vi "Main_Timing.vi"() -> ()   [LabVIEW 2012]
panel:
  in  "Wait between operations (ms)":dbl
  in  "Input Expression":string
  out "While Iterations":i32
  out "Elapsed Time (ms)":dbl caption="Elapsed Time (s)"
  in  "Time Target (ms)":dbl=5.0 caption="Time Target (s)"
  # "(5 operations)"
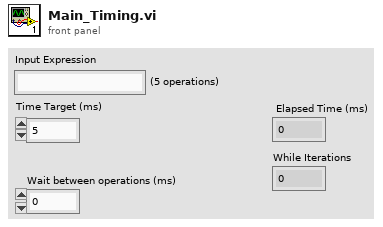
[diagram p1: front panel]
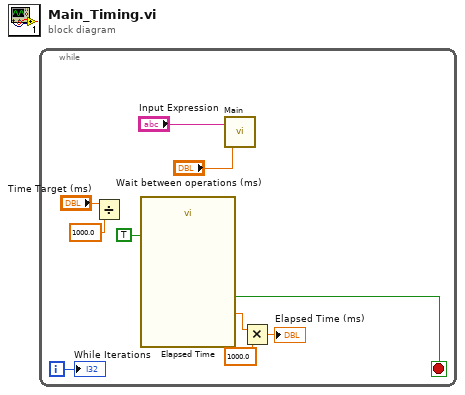
[diagram p0: block diagram]
diagram:
  n1 = while {
    i -> [w8]
    stop <- w9 stop-if-true
    n2 = Divide(x="Time Target (ms)", y=1000.0) -> ()  [unwired: 1 out]
    n3 = call "Elapsed Time"("Auto Reset"=TRUE) -> ("Elapsed Time (s)"=w3:dbl, "Time has Elapsed"=w9:bool)  [unwired: 11 in, 6 out]
    n4 = call "Main.vi"("Wait (ms)"="Wait between operations (ms)", "Input Expression"="Input Expression") -> ()  [unwired: 1 out]
    n5 = Multiply(x=w3, y=1000.0) -> (x*y=→"Elapsed Time (ms)":dbl)
    "While Iterations" <- w8
  }
